vi "Auto_Drive (2).vi"(10 "Target":dbl=40.0 format="%#_13g", 11 "Drive Effort":dbl=0.1) -> ()   [LabVIEW 2016]
uses:
  <vilib>/Rock Robotics/WPI/SafetyOutput/WPI_SafetyOutputConfigMenu.ctl
  Global 2.vi
panel:
  in  "kP":dbl=0.35 format="%#_13g"
  in  "kD":dbl=1.6 format="%#_13g"
  in  "Scaling Factor":dbl=16.0 format="%#_13g"
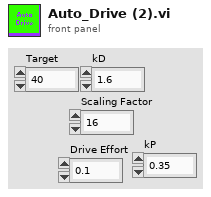
[diagram p1: front panel]
types:
  T1 = typedef "WPI_SafetyOutputConfigMenu.ctl" = enum16{"Enable", "Disable"}
  T2 = typedef "WPI_MotorControlDeviceRef.ctl" = cluster{"DeviceStatus":errorcluster, "Type":T3, "PWM":cluster{"PWM Channel":T4, "DeadBand":T5}, "CAN":cluster{"Device Number":u8, "SetOutput VI Ref":variant, "GetOutput VI Ref":variant, "Enable VI Ref":variant, "Disable VI Ref":variant, "Data":variant}, "Invert":bool}
  T3 = typedef "WPI_MotorControlType.ctl" = enum16{"PWM", "CAN"}
  T4 = typedef "FPGA_DIOPWMChannel.ctl" = enum8{"PWM 0", "PWM 1", "PWM 2", "PWM 3", "PWM 4", "PWM 5", "PWM 6", "PWM 7", "PWM 8", "PWM 9", "PWM MXP 0", "PWM MXP 1", "PWM MXP 2", "PWM MXP 3", "PWM MXP 4", "PWM MXP 5", "PWM MXP 6", "PWM MXP 7", "PWM MXP 8", "PWM MXP 9", "Invalid"}
  T5 = typedef "WPI_PWMDeadband.ctl" = cluster{"Name":string, "maxPositivePwm":i32, "minPositivePwm":i32, "centerPwm":i32, "maxNegativePwm":i32, "minNegativePwm":i32, "angularRange":u16}
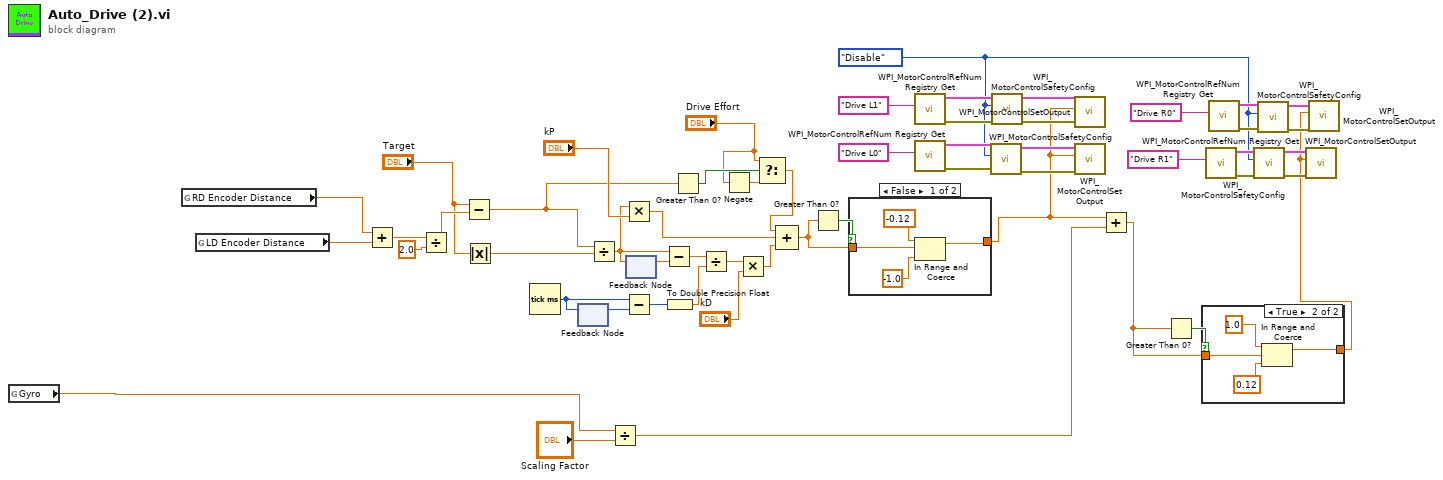
[diagram p0: block diagram]
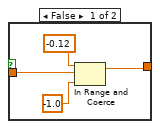
[diagram p2: hidden frame]
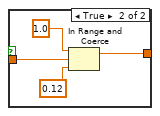
[diagram p3: hidden frame]
diagram:
  w34 = WPI_SafetyOutputConfigMenu."Disable" ("mode")
  n1 = global read "Global 2.vi" "Gyro"() -> (w31:dbl)
  n2 = global read "Global 2.vi" "RD Encoder Distance"() -> (w11:dbl)
  n3 = global read "Global 2.vi" "LD Encoder Distance"() -> (w12:dbl)
  n4 = Add(x=w11, y=w12) -> (x+y=w30:dbl)
  n5 = Divide(x=w30, y=2.0) -> (x/y=w28:dbl)
  n6 = Subtract(x="Target", y=w28) -> (x-y=w5:dbl)
  n7 = Absolute Value(x="Target") -> (abs(x)=w7:dbl)
  n8 = Tick Count (ms)() -> (millisecond timer value=w24:u32)
  n9 = feedback #1() -> (w25:u32)  [unwired: 1 in]
  n10 = feedback-in #1(w24) -> ()
  n11 = Divide(x=w5, y=w7) -> (x/y=w6:dbl)
  n12 = Divide(x=w31, y="Scaling Factor") -> (x/y=w32:dbl)
  n13 = Multiply(x=w6, y="kP") -> (x*y=w18:dbl)
  n14 = Subtract(x=w24, y=w25) -> (x-y=w22:u32)
  n15 = feedback #2() -> (w26:dbl)  [unwired: 1 in]
  n16 = feedback-in #2(w6) -> ()
  n17 = Subtract(x=w6, y=w26) -> (x-y=w23:dbl)
  n18 = To Double Precision Float(number=w22) -> (double precision float=w21:dbl)
  n19 = Greater Than 0?(x=w5) -> (x > 0?=w4:bool)
  n20 = Divide(x=w23, y=w21) -> (x/y=w20:dbl)
  n21 = Negate(x="Drive Effort") -> (-x=w3:dbl)
  n22 = Multiply(x=w20, y="kD") -> (x*y=w17:dbl)
  n23 = Select(t="Drive Effort", s=w4, f=w3) -> (s? t:f=w1:dbl)
  n24 = Compound Arithmetic op=ADD(w1, w18, w17) -> (w15:dbl)
  n25 = Greater Than 0?(x=w15) -> (x > 0?=w16:bool)
  n26 = case shown="False" w16 {
    tunnel: [w55 w60] -> w14
    tunnel: w15 -> [w56 w59]
    frame False {
      n27 = In Range and Coerce(upper limit=-0.12, x=w56, lower limit=-1.0) -> (coerced(x)=w55:dbl)  [unwired: 1 out]
    }
    frame True {
      n28 = In Range and Coerce(upper limit=1.0, x=w59, lower limit=0.12) -> (coerced(x)=w60:dbl)  [unwired: 1 out]
    }
  }
  n29 = call <vilib>:"WPI_MotorControlRefNum Registry Get.vi"("refnum name"="Drive L1") -> ("error out"=w49:errorcluster, "MotorControlDevRef"=w50:T2)  [unwired: 9 in]
  n30 = call <vilib>:"WPI_MotorControlRefNum Registry Get.vi"("refnum name"="Drive L0") -> ("error out"=w45:errorcluster, "MotorControlDevRef"=w46:T2)  [unwired: 9 in]
  n31 = call <vilib>:"WPI_MotorControlSafetyConfig.vi"("error in (no error)"=w45, "mode"=w34, "MotorControlDevRef"=w46) -> ("error out"=w43:errorcluster, "MotorControlDevRef"=w44:T2)  [unwired: 7 in]
  n32 = call <vilib>:"WPI_MotorControlSafetyConfig.vi"("error in (no error)"=w49, "mode"=w34, "MotorControlDevRef"=w50) -> ("error out"=w47:errorcluster, "MotorControlDevRef"=w48:T2)  [unwired: 7 in]
  n33 = call <vilib>:"WPI_MotorControlSetOutput.vi"("error in (no error)"=w47, "Output"=w14, "MotorControlDevRef"=w48) -> ()  [unwired: 6 in, 3 out]
  n34 = call <vilib>:"WPI_MotorControlSetOutput.vi"("error in (no error)"=w43, "Output"=w14, "MotorControlDevRef"=w44) -> ()  [unwired: 6 in, 3 out]
  n35 = Add(x=w14, y=w32) -> (x+y=w8:dbl)
  n36 = Greater Than 0?(x=w8) -> (x > 0?=w10:bool)
  n37 = case shown="True" w10 {
    tunnel: [w63 w68] -> w9
    tunnel: w8 -> [w64 w67]
    frame False {
      n38 = In Range and Coerce(upper limit=-0.12, x=w64, lower limit=-1.0) -> (coerced(x)=w63:dbl)  [unwired: 1 out]
    }
    frame True {
      n39 = In Range and Coerce(upper limit=1.0, x=w67, lower limit=0.12) -> (coerced(x)=w68:dbl)  [unwired: 1 out]
    }
  }
  n40 = call <vilib>:"WPI_MotorControlRefNum Registry Get.vi"("refnum name"="Drive R1") -> ("error out"=w37:errorcluster, "MotorControlDevRef"=w38:T2)  [unwired: 9 in]
  n41 = call <vilib>:"WPI_MotorControlRefNum Registry Get.vi"("refnum name"="Drive R0") -> ("error out"=w41:errorcluster, "MotorControlDevRef"=w42:T2)  [unwired: 9 in]
  n42 = call <vilib>:"WPI_MotorControlSafetyConfig.vi"("error in (no error)"=w37, "mode"=w34, "MotorControlDevRef"=w38) -> ("error out"=w36:errorcluster, "MotorControlDevRef"=w35:T2)  [unwired: 7 in]
  n43 = call <vilib>:"WPI_MotorControlSafetyConfig.vi"("error in (no error)"=w41, "mode"=w34, "MotorControlDevRef"=w42) -> ("error out"=w40:errorcluster, "MotorControlDevRef"=w39:T2)  [unwired: 7 in]
  n44 = call <vilib>:"WPI_MotorControlSetOutput.vi"("error in (no error)"=w36, "Output"=w9, "MotorControlDevRef"=w35) -> ()  [unwired: 6 in, 3 out]
  n45 = call <vilib>:"WPI_MotorControlSetOutput.vi"("error in (no error)"=w40, "Output"=w9, "MotorControlDevRef"=w39) -> ()  [unwired: 6 in, 3 out]
